vi "Get configuration Address.vi"(1 "文件名":string="myDAQConfi.ini") -> (0 "配置文件路径":path)   [LabVIEW 2016]
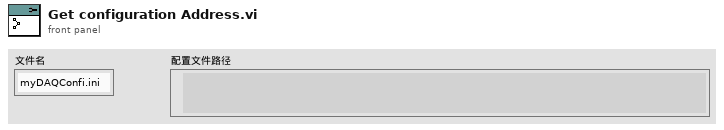
[diagram p1: front panel]
types:
  T1 = enum32{"invalid app kind", "Development System", "Run Time System", "Student Edition", "Embedded LabVIEW", "Evaluation", "Custom"}
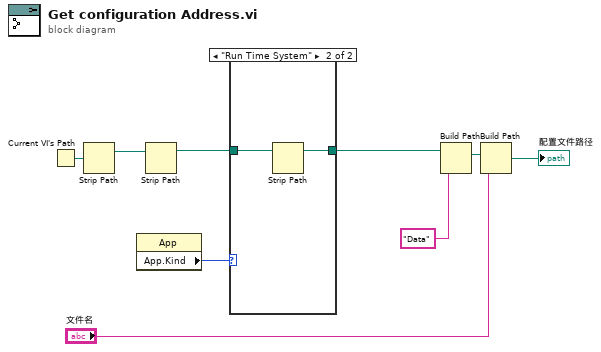
[diagram p0: block diagram]
diagram:
  n1 = Current VI's Path() -> (path=w9:path)
  n2 = Strip Path(path=w9) -> (stripped path=w3:path)  [unwired: 1 out]
  n3 = property class="App"() -> ("App.Kind"=w7:T1)  [unwired: 2 in, 2 out]
  n4 = Strip Path(path=w3) -> (stripped path=w2:path)  [unwired: 1 out]
  n5 = case shown="\"Run Time System\"" w7 {
    tunnel: w2 -> [w10 w12]
    tunnel: [w10 w11] -> w6
    frame "invalid app kind", Default {
    }
    frame "Run Time System" {
      n6 = Strip Path(path=w12) -> (stripped path=w11:path)  [unwired: 1 out]
    }
  }
  n7 = Build Path(base path=w6, name or relative path="Data" ("名称或相对路径")) -> (appended path=w5:path)
  n8 = Build Path(base path=w5, name or relative path="文件名") -> (appended path=→"配置文件路径":path)
